vi "Set Grating.vi"(8 "error in (no error)":errorcluster, 10 "Grating ID":i32, 11 "SpectraPro in":refnum<class "SpectraPro.lvclass">) -> (0 "error out":errorcluster, 2 "Grating ID out":i32, 3 "SpectraPro out":refnum<class "SpectraPro.lvclass">)   [LabVIEW 2019, in "SpectraPro.lvclass"]
uses:
  SpectraPro.lvclass
  SpectraPro.lvclass/SpectraPro.ctl
  SpectraPro-LabVIEW-Driver/SpectraPro.lvlib
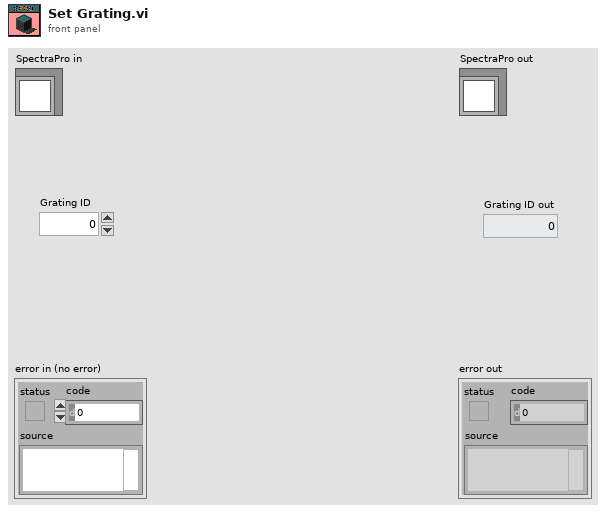
[diagram p1: front panel]
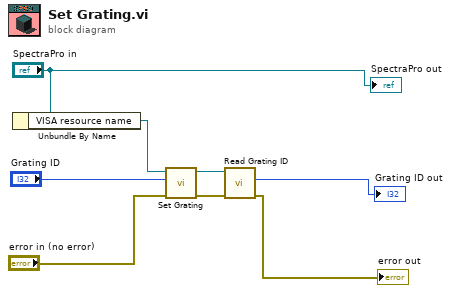
[diagram p0: block diagram]
diagram:
  n1 = Unbundle By Name("SpectraPro in") -> ("VISA resource name"=w7:refnum<visa-resource-name>)
  n2 = call "Set Grating.vi"("error in (no error)"="error in (no error)", "Grating ID"="Grating ID", "VISA resource name"=w7) -> ("error out"=w5:errorcluster, "VISA resource name out"=w4:refnum<visa-resource-name>)  [unwired: 6 in, 1 out]
  n3 = call "Read Grating ID.vi"("error in (no error)"=w5, "VISA resource name"=w4) -> ("error out"=→"error out":errorcluster, "Grating ID"=→"Grating ID out":i32)  [unwired: 6 in, 2 out]
  "SpectraPro out" <- "SpectraPro in"
